vi "Copy Image to Pixmap (ARGB with Mask).vi"(7 "Pixmap Offset (Default 0,0)":T2, 8 "error in (no error)":errorcluster, 10 "Greyscale Mask":T1, 11 "ARGB Image Source":T4) -> (0 "error out":errorcluster, 3 "Pixmap Image Data":T3)   [LabVIEW 2020, in "image.lvlib"]
uses:
  image.lvlib
  ARGB Image.ctl
  <vilib>/picture/picture.llb/imagedata.ctl
  Image Draw Offset.ctl
  Greyscale Image.ctl
  5c639587-cf36-4d54-93d9-e654c7c24c6e.vi
  common/Module Path.vi
  <vilib>/Utility/error.llb/Error Cluster From Error Code.vi
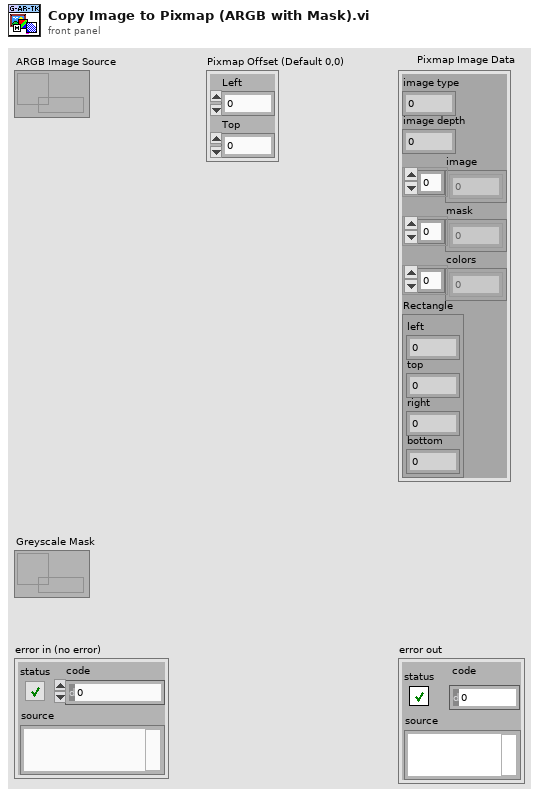
[diagram p1: front panel]
types:
  T1 = typedef "image.lvlib/Greyscale Image.ctl" = refnum<data-value>
  T2 = typedef "image.lvlib/Image Draw Offset.ctl" = cluster{"Left":i16, "Top":i16}
  T3 = typedef "imagedata.ctl" = cluster{"image type":i32, "image depth":i32, "image":u8[], "mask":u8[], "colors":u32[], "Rectangle":cluster{"left":i16, "top":i16, "right":i16, "bottom":i16}}
  T4 = typedef "image.lvlib/ARGB Image.ctl" = refnum<data-value>
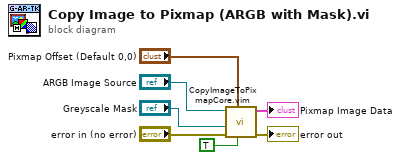
[diagram p0: block diagram]
diagram:
  n1 = call "CopyImageToPixmapCore.vim"("Has Mask"=TRUE, "Pixmap Offset (Default 0,0)"="Pixmap Offset (Default 0,0)", "error in (no error)"="error in (no error)", "Mask Image"="Greyscale Mask", "Destination Image"="ARGB Image Source") -> ("error out"=→"error out":errorcluster, "Pixmap"=→"Pixmap Image Data":T3)  [unwired: 5 in]
